vi "Start Section.vi"(8 "error in (no error)":errorcluster {"code" format="Error %.0f"}, 10 "Section":string, 11 "UI Interaction in":refnum<class "UI Interaction.lvclass">) -> (0 "error out":errorcluster {"code" format="Error %.0f"}, 3 "UI Interaction out":refnum<class "UI Interaction.lvclass">)   [LabVIEW 2023, in "UI Interaction.lvclass"]
uses:
  UI Interaction.lvclass
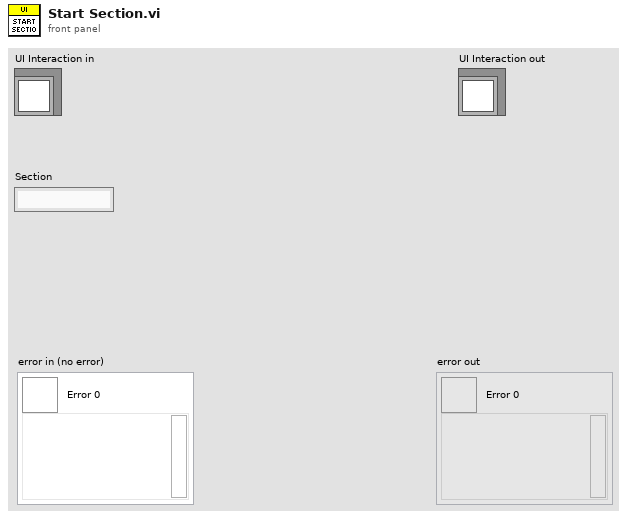
[diagram p1: front panel]
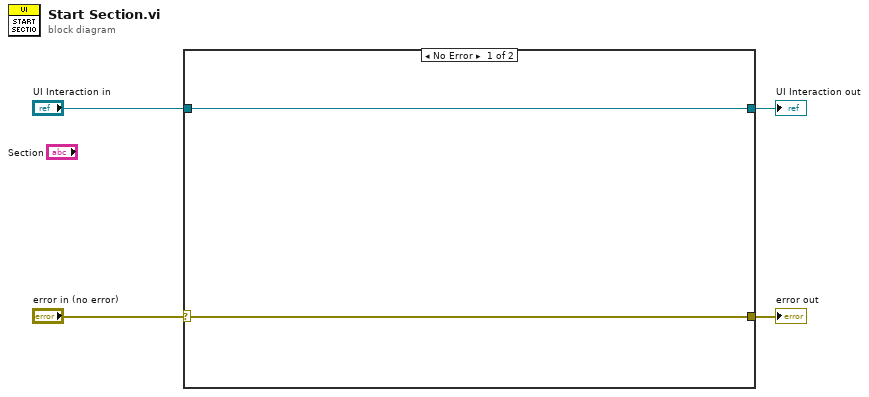
[diagram p0: block diagram]
diagram:
  n1 = case shown="No Error" "error in (no error)" {
    selector: "error in (no error)" -> [w5 w8]
    tunnel: [w5 w8] -> w3
    tunnel: [w6 w7] -> w1
    tunnel: "UI Interaction in" -> [w6 w7]
    frame No Error {
    }
    frame Error {
    }
  }
  "error out" <- w3
  "UI Interaction out" <- w1
